vi "ShootAndTransfer5.vi"() -> ()   [LabVIEW 2010]
uses:
  EDSDK-Labview.llb/kEdsObjectEvents.ctl
  EDSDK-Labview.llb/LVuserEventForEDS.ctl
  EDSDK-Labview.llb/kEdsImageSrcs.ctl
  EDSDK-Labview.llb/EdsImageInfo.ctl
  EDSDK-Labview.llb/kEdsProperties.ctl
  EDSDK-Labview.llb/kEdsCameraStatusCommands.ctl
  EDSDK-Labview.llb/kEdsCameraCommands.ctl
  kernel32.dll
  EDSDK-Labview.llb/kEdsCameraCommand_ShutterButton.ctl
panel:
  out "images to download":i32
  out "images to decode":i32
  out "dt download":u32[](array[numeric])
  out "delay from shoot":u32[](array[numeric])
  out "dt decode":u32[](array[numeric])
  out "total decode cycle":u32
  out "body ids":u32[](array[numeric])
  out "ref":u32
  out "grab error out":errorcluster
  out "shoot error out":errorcluster
  in  "shoot cycle duration":u32=4000
  out "images":T1[](array[plugin-control])
  out "shoot #":i32
  out "event":T2 items=["All"=512, "VolumeInfoChanged"=513, "VolumeUpdateItems"=514, "FolderUpdateItems"=515, "DirItemCreated"=516, "DirItemRemoved"=517, "DirItemInfoChanged"=518, "DirItemContentChanged"=519, "DirItemRequestTransfer"=520, "DirItemRequestTransferDT"=521, "DirItemCancelTransferDT"=522, "VolumeAdded"=524, "VolumeRemoved"=525]
  in  "Image Type":T3=4 items=["Grayscale (U8)", "Grayscale (I16)", "Grayscale (SGL)", "Complex (CSG)", "RGB (U32)", "HSL (U32)", "RGB (U64)", "Grayscale (U16)"]
  in  "stop":bool
  out "cameras":u32
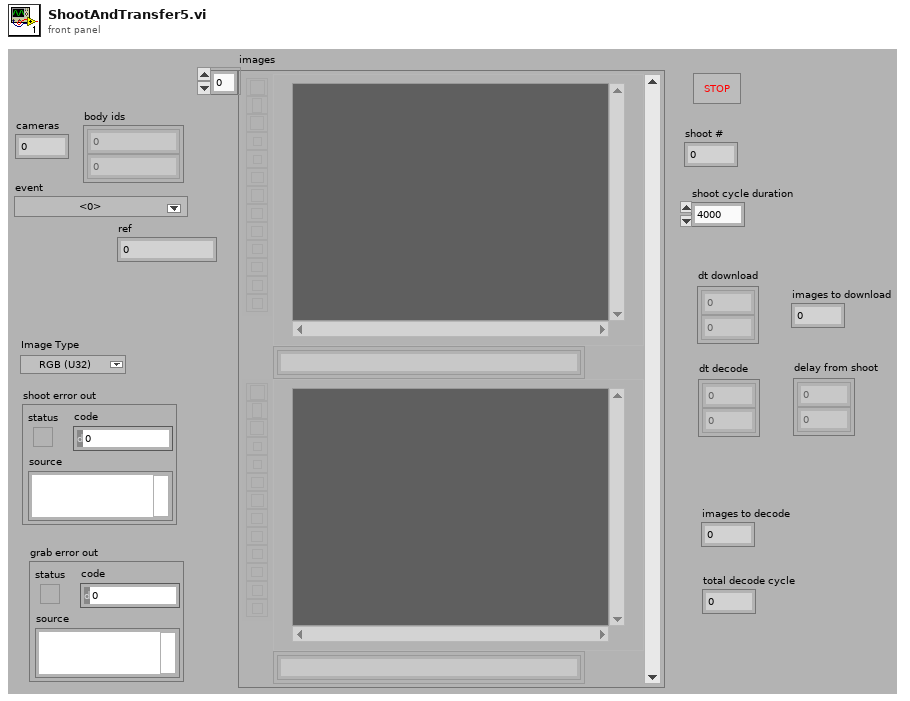
[diagram p1: front panel]
types:
  T1 = typedef "IMAQ Image.ctl" = refnum<image>
  T2 = typedef "kEdsObjectEvents.ctl" = u32
  T3 = typedef "Image Type" = u32
  T4 = typedef "LVuserEventForEDS.ctl" = cluster{"LVUserEventRef":u32, "event":u32, "ref":u32}
  T5 = typedef "kEdsImageSrcs.ctl" = u32
  T6 = typedef "EdsImageInfo.ctl" = cluster{"width":u32, "height":u32, "# components":u32, "bit depth":u32, "rect":u32[], "reserved 1":u32, "reserved 2":u32}
  T7 = cluster{"time Request":u32, "time downloaded":u32, "ImageRef":u32, "ImageSource":T5, "StreamRef":u32, "ImageInfo":T6}
  T8 = cluster{"numberOfFreeClusters":i32, "numberOfFreeSectors":i32, "reset":bool}
  T9 = typedef "kEdsProperties.ctl" = u32
  T10 = typedef "kEdsCameraCommands.ctl" = u32
  T11 = typedef "kEdsCameraCommand_ShutterButton.ctl" = u32
  T12 = cluster{"time":u32, "timer after download":u32, "ImageRef":u32, "ImageSource":T5, "outStreamRef":u32, "outImageInfo":T6}
  T13 = typedef "kEdsCameraStatusCommands.ctl" = u32
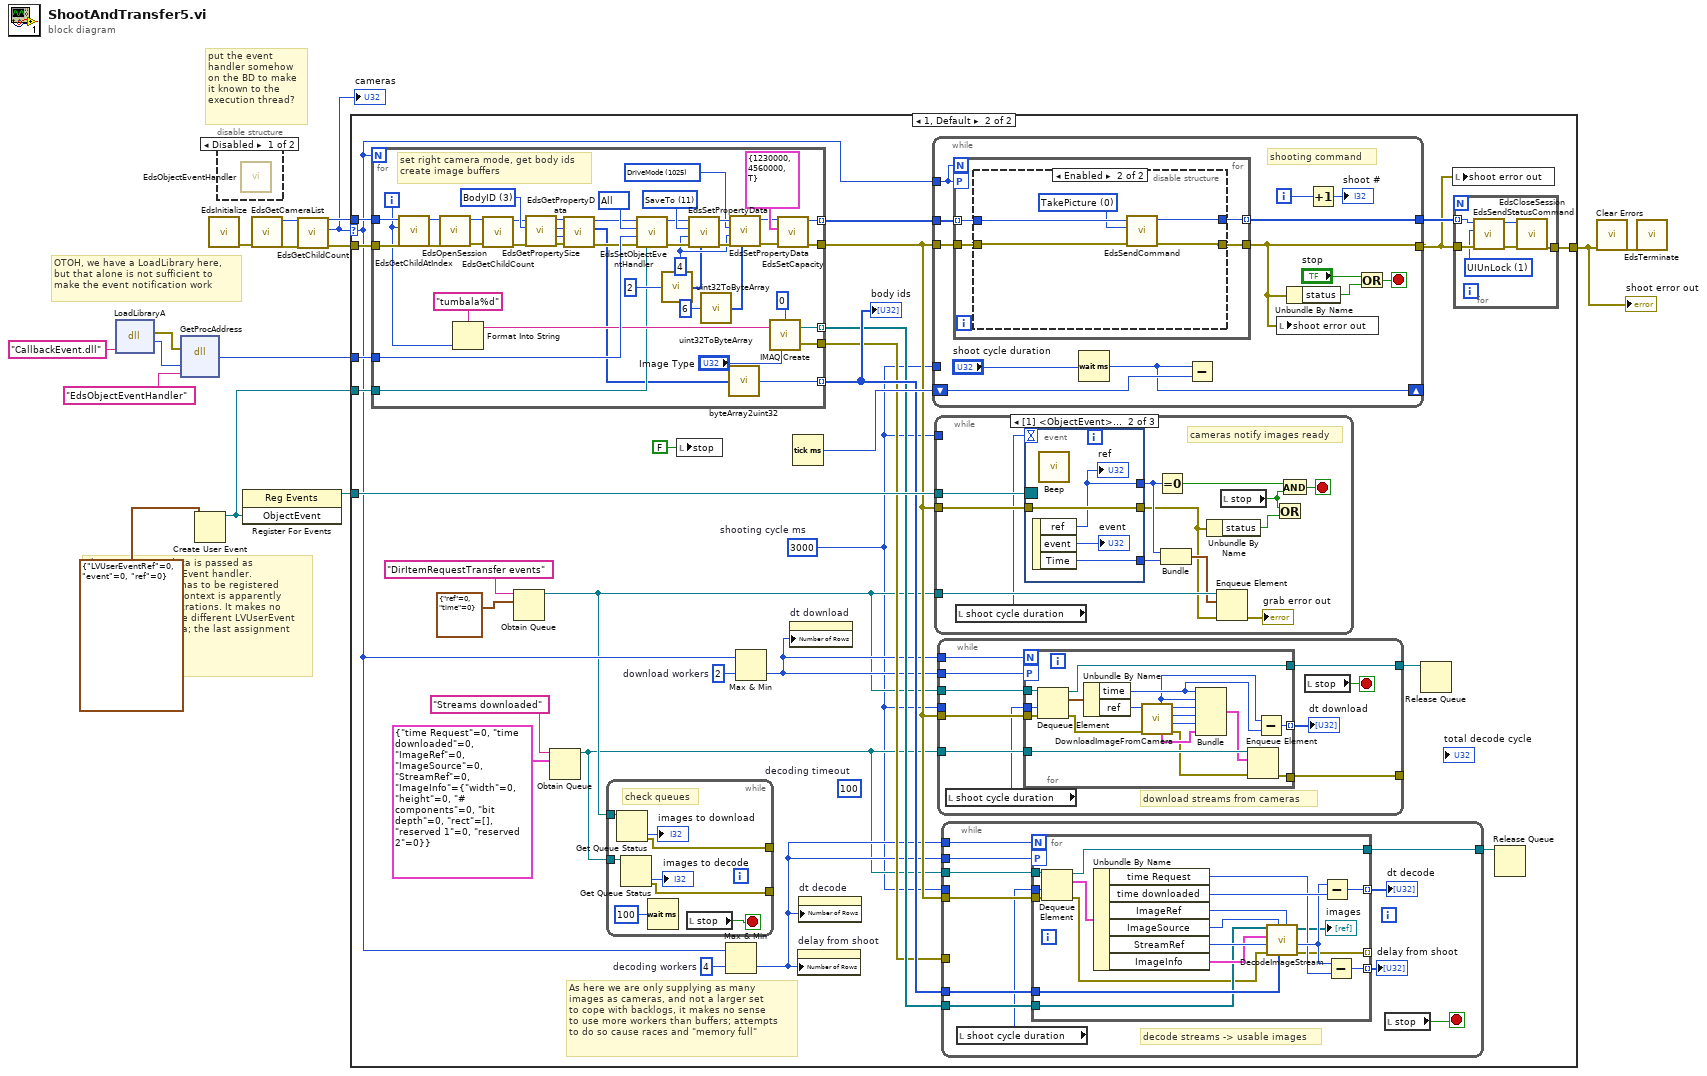
[diagram p0: block diagram]
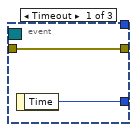
[diagram p4: hidden frame]
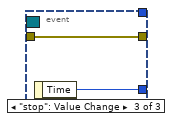
[diagram p5: hidden frame]
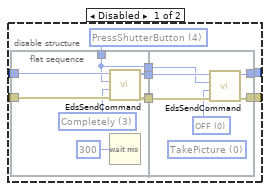
[diagram p6: hidden frame]
diagram:
  # "The LVUserEvent data is passed as \nInContext to EDSSetEvent handler.\nEven if the callback has to be registered\nfor each camera, InContext is apparently\ncommon to all registrations. It makes no\nsense to try to define different LVUserEvent\ndata for each camera; the last assignment\nrules."
  # "OTOH, we have a LoadLibrary here,\nbut that alone is not sufficient to\nmake the event notification work"
  # "put the event\nhandler somehow\non the BD to make\nit known to the\nexecution thread?"
  n1 = dll-call lib="kernel32.dll" fn="LoadLibraryA"("libraryName"="CallbackEvent.dll") -> (error out=w7:errorcluster, "return type"=w10:u32)  [unwired: 4 in, 1 out]
  n2 = dll-call lib="kernel32.dll" fn="GetProcAddress"(error in=w7, "address"=w10, "procName"="EdsObjectEventHandler") -> ("return type"=w8:u32)  [unwired: 4 in, 2 out]
  n3 = Create User Event(user event datatype=T4 {"LVUserEventRef"=0, "event"=0, "ref"=0} ("ObjectEvent")) -> (user event=w2:refnum<user-event>)  [unwired: 1 in, 1 out]
  n4 = call "EdsInitialize.vi"() -> ("error out"=w5:errorcluster)  [unwired: 11 in]
  n5 = disable-structure shown="Disabled" {
    frame Disabled {
      n6 = call "EdsObjectEventHandler.vi"() -> ()  [unwired: 7 in, 2 out]
    }
    frame Enabled {
    }
  }
  n7 = register-events(w2) -> (reference out=w3:refnum<event-registration>)  [unwired: 2 in, 1 out]
  n8 = call "EdsGetCameraList.vi"("error in"=w5) -> ("error out"=w14:errorcluster, "outCameraListRef"=w1:u32)  [unwired: 9 in]
  n9 = call "EdsGetChildCount.vi"("error in"=w14, "inRef"=w1) -> ("error out"=w6:errorcluster, "count"=w12:u32, "inRef dup"=w13:u32)  [unwired: 7 in]
  "cameras" <- w12
  n10 = case shown="1, Default" w12 {
    selector: w12 -> [_ w23]
    tunnel: w13 -> [_ w46]
    tunnel: w6 -> [w17 w45]
    tunnel: [w17 w44] -> w15
    tunnel: w8 -> [_ w43]
    tunnel: w3 -> [_ w37]
    tunnel: w2 -> [_ w36]
    frame 0 {
    }
    frame 1, Default {
      (unwired) u32 100  # decoding timeout
      w24 = u32 2  # download workers
      w22 = u32 4  # decoding workers
      w18 = u32 3000  # shooting cycle ms
      # "As here we are only supplying as many\nimages as cameras, and not a larger set\nto cope with backlogs, it makes no sense\nto use more workers than buffers; attempts\nto do so cause races and \"memory full\""
      n11 = for {
        N: w23 -> [_]
        tunnel: w46 -> [w180]
        tunnel: w45 -> [w179]
        tunnel: [w174] -> w27 mode=indexing
        tunnel: [w173] -> w26
        tunnel: w43 -> [w170]
        tunnel: [w152] -> w39 mode=indexing
        tunnel: [w151] -> w31
        tunnel: w36 -> [w153]
        tunnel: [w140] -> w28 mode=indexing
        i -> [w156]
        w147 = T9 3 items=["Unknown"=65535, "ProductName"=2, "BodyID"=3, "OwnerName"=4, "MakerName"=5, "DateTime"=6, "FirmwareVersion"=7, "BatteryLevel"=8, "CFn"=9, "SaveTo"=11, "CurrentStorage"=12, "CurrentFolder"=13, "MyMenu"=14, "BatteryQuality"=16, "HDDirectoryStructure"=32, "ImageQuality"=256, "JpegQuality"=257, "Orientation"=258, "ICCProfile"=259, "FocusInfo"=260, "DigitalExposure"=261, "WhiteBalance"=262, "ColorTemperature"=263, "WhiteBalanceShift"=264, "Contrast"=265, "ColorSaturation"=266, "ColorTone"=267, "Sharpness"=268, "ColorSpace"=269, "ToneCurve"=270, "PhotoEffect"=271, "FilterEffect"=272, "ToningEffect"=273, "ParameterSet"=274, "ColorMatrix"=275, "PictureStyle"=276, "PictureStyleDesc"=277, "ETTL2Mode"=279, "PictureStyleCaption"=512, "Linear"=768, "ClickWBPoint"=769, "WBCoeffs"=770, "GPSVersionID"=2048, "GPSLatitudeRef"=2049, "GPSLatitude"=2050, "GPSLongitudeRef"=2051, "GPSLongitude"=2052, "GPSAltitudeRef"=2053, "GPSAltitude"=2054, "GPSTimeStamp"=2055, "GPSSatellites"=2056, "GPSStatus"=2057, "GPSMapDatum"=2066, "GPSDateStamp"=2077, "AtCapture_Flag"=2147483648, "AEMode"=1024, "DriveMode"=1025, "ISOSpeed"=1026, "MeteringMode"=1027, "AFMode"=1028, "Av"=1029, "Tv"=1030, "ExposureCompensation"=1031, "FlashCompensation"=1032, "FocalLength"=1033, "AvailableShots"=1034, "Bracket"=1035, "WhiteBalanceBracket"=1036, "LensName"=1037, "AEBracket"=1038, "FEBracket"=1039, "ISOBracket"=1040, "NoiseReduction"=1041, "FlashOn"=1042, "RedEye"=1043, "FlashMode"=1044, "LensStatus"=1046, "Artist"=1048, "Copyright"=1049, "DepthOfField"=1051, "EFCompensation"=1054, "Evf_OutputDevice"=1280, "Evf_Mode"=1281, "Evf_WhiteBalance"=1282, "Evf_ColorTemperature"=1283, "Evf_DepthOfFieldPreview"=1284, "Evf_Zoom"=1287, "Evf_ZoomPosition"=1288, "Evf_FocusAid"=1289, "Evf_Histogram"=1290, "Evf_ImagePosition"=1291, "Evf_HistogramStatus"=1292, "Evf_AFMode"=1294, "Evf_CoordinateSystem"=1344, "Evf_ZoomRect"=1345] ("inPropertyID")
        w161 = T9 1025 items=["Unknown"=65535, "ProductName"=2, "BodyID"=3, "OwnerName"=4, "MakerName"=5, "DateTime"=6, "FirmwareVersion"=7, "BatteryLevel"=8, "CFn"=9, "SaveTo"=11, "CurrentStorage"=12, "CurrentFolder"=13, "MyMenu"=14, "BatteryQuality"=16, "HDDirectoryStructure"=32, "ImageQuality"=256, "JpegQuality"=257, "Orientation"=258, "ICCProfile"=259, "FocusInfo"=260, "DigitalExposure"=261, "WhiteBalance"=262, "ColorTemperature"=263, "WhiteBalanceShift"=264, "Contrast"=265, "ColorSaturation"=266, "ColorTone"=267, "Sharpness"=268, "ColorSpace"=269, "ToneCurve"=270, "PhotoEffect"=271, "FilterEffect"=272, "ToningEffect"=273, "ParameterSet"=274, "ColorMatrix"=275, "PictureStyle"=276, "PictureStyleDesc"=277, "ETTL2Mode"=279, "PictureStyleCaption"=512, "Linear"=768, "ClickWBPoint"=769, "WBCoeffs"=770, "GPSVersionID"=2048, "GPSLatitudeRef"=2049, "GPSLatitude"=2050, "GPSLongitudeRef"=2051, "GPSLongitude"=2052, "GPSAltitudeRef"=2053, "GPSAltitude"=2054, "GPSTimeStamp"=2055, "GPSSatellites"=2056, "GPSStatus"=2057, "GPSMapDatum"=2066, "GPSDateStamp"=2077, "AtCapture_Flag"=2147483648, "AEMode"=1024, "DriveMode"=1025, "ISOSpeed"=1026, "MeteringMode"=1027, "AFMode"=1028, "Av"=1029, "Tv"=1030, "ExposureCompensation"=1031, "FlashCompensation"=1032, "FocalLength"=1033, "AvailableShots"=1034, "Bracket"=1035, "WhiteBalanceBracket"=1036, "LensName"=1037, "AEBracket"=1038, "FEBracket"=1039, "ISOBracket"=1040, "NoiseReduction"=1041, "FlashOn"=1042, "RedEye"=1043, "FlashMode"=1044, "LensStatus"=1046, "Artist"=1048, "Copyright"=1049, "DepthOfField"=1051, "EFCompensation"=1054, "Evf_OutputDevice"=1280, "Evf_Mode"=1281, "Evf_WhiteBalance"=1282, "Evf_ColorTemperature"=1283, "Evf_DepthOfFieldPreview"=1284, "Evf_Zoom"=1287, "Evf_ZoomPosition"=1288, "Evf_FocusAid"=1289, "Evf_Histogram"=1290, "Evf_ImagePosition"=1291, "Evf_HistogramStatus"=1292, "Evf_AFMode"=1294, "Evf_CoordinateSystem"=1344, "Evf_ZoomRect"=1345] ("inPropertyID")
        w171 = T2 512 items=["All"=512, "VolumeInfoChanged"=513, "VolumeUpdateItems"=514, "FolderUpdateItems"=515, "DirItemCreated"=516, "DirItemRemoved"=517, "DirItemInfoChanged"=518, "DirItemContentChanged"=519, "DirItemRequestTransfer"=520, "DirItemRequestTransferDT"=521, "DirItemCancelTransferDT"=522, "VolumeAdded"=524, "VolumeRemoved"=525] ("inEvent")
        w162 = u32 4 ("inPropertySize")
        w172 = T9 11 items=["Unknown"=65535, "ProductName"=2, "BodyID"=3, "OwnerName"=4, "MakerName"=5, "DateTime"=6, "FirmwareVersion"=7, "BatteryLevel"=8, "CFn"=9, "SaveTo"=11, "CurrentStorage"=12, "CurrentFolder"=13, "MyMenu"=14, "BatteryQuality"=16, "HDDirectoryStructure"=32, "ImageQuality"=256, "JpegQuality"=257, "Orientation"=258, "ICCProfile"=259, "FocusInfo"=260, "DigitalExposure"=261, "WhiteBalance"=262, "ColorTemperature"=263, "WhiteBalanceShift"=264, "Contrast"=265, "ColorSaturation"=266, "ColorTone"=267, "Sharpness"=268, "ColorSpace"=269, "ToneCurve"=270, "PhotoEffect"=271, "FilterEffect"=272, "ToningEffect"=273, "ParameterSet"=274, "ColorMatrix"=275, "PictureStyle"=276, "PictureStyleDesc"=277, "ETTL2Mode"=279, "PictureStyleCaption"=512, "Linear"=768, "ClickWBPoint"=769, "WBCoeffs"=770, "GPSVersionID"=2048, "GPSLatitudeRef"=2049, "GPSLatitude"=2050, "GPSLongitudeRef"=2051, "GPSLongitude"=2052, "GPSAltitudeRef"=2053, "GPSAltitude"=2054, "GPSTimeStamp"=2055, "GPSSatellites"=2056, "GPSStatus"=2057, "GPSMapDatum"=2066, "GPSDateStamp"=2077, "AtCapture_Flag"=2147483648, "AEMode"=1024, "DriveMode"=1025, "ISOSpeed"=1026, "MeteringMode"=1027, "AFMode"=1028, "Av"=1029, "Tv"=1030, "ExposureCompensation"=1031, "FlashCompensation"=1032, "FocalLength"=1033, "AvailableShots"=1034, "Bracket"=1035, "WhiteBalanceBracket"=1036, "LensName"=1037, "AEBracket"=1038, "FEBracket"=1039, "ISOBracket"=1040, "NoiseReduction"=1041, "FlashOn"=1042, "RedEye"=1043, "FlashMode"=1044, "LensStatus"=1046, "Artist"=1048, "Copyright"=1049, "DepthOfField"=1051, "EFCompensation"=1054, "Evf_OutputDevice"=1280, "Evf_Mode"=1281, "Evf_WhiteBalance"=1282, "Evf_ColorTemperature"=1283, "Evf_DepthOfFieldPreview"=1284, "Evf_Zoom"=1287, "Evf_ZoomPosition"=1288, "Evf_FocusAid"=1289, "Evf_Histogram"=1290, "Evf_ImagePosition"=1291, "Evf_HistogramStatus"=1292, "Evf_AFMode"=1294, "Evf_CoordinateSystem"=1344, "Evf_ZoomRect"=1345] ("inPropertyID")
        # "set right camera mode, get body ids\ncreate image buffers"
        n12 = call "EdsGetChildAtIndex.vi"("error in"=w179, "index"=w156, "inRef"=w180) -> ("error out"=w181:errorcluster, "outRef"=w182:u32)  [unwired: 7 in]
        n13 = call "EdsOpenSession.vi"("error in"=w181, "inCameraRef"=w182) -> ("error out"=w177:errorcluster, "inCameraRef dup"=w178:u32)  [unwired: 8 in]
        n14 = Format Into String(format string="tumbala%d" ("Image Name"), w156) -> (resulting string=w154:string)  [unwired: 2 in, 1 out]
        n15 = call "EdsGetChildCount.vi"("error in"=w177, "inRef"=w178) -> ("error out"=w145:errorcluster, "inRef dup"=w144:u32)  [unwired: 7 in, 1 out]
        n16 = call "EdsGetPropertySize.vi"("error in"=w145, "inPropertyID"=w147, "inRef"=w144) -> ("error out"=w149:errorcluster, "outSize"=w148:u32, "inPropertyID dup"=w150:T9, "inRef dup"=w146:u32)  [unwired: 4 in, 1 out]
        n17 = call "EdsGetPropertyData.vi"("error in"=w149, "inPropertySize"=w148, "inPropertyID"=w150, "inRef"=w146) -> ("error out"=w143:errorcluster, "outPropertyData"=w141:u8[], "inRef dup"=w142:u32)  [unwired: 5 in]
        n18 = call "EdsSetObjectEventHandler.vi"("user event out"=w153, "error in"=w143, "inObjectEventHandler"=w170, "inEvent"=w171, "inCameraRef"=w142) -> ("error out"=w169:errorcluster, "inCameraRef dup"=w168:u32)  [unwired: 2 in]
        n19 = call "uint32ToByteArray.vi"("Numeric"=u32 2) -> ("inPropertyData"=w160:u8[])  [unwired: 4 in]
        n20 = call "EdsSetPropertyData.vi"("inPropertyData"=w160, "error in"=w169, "inPropertySize"=w162, "inPropertyID"=w172, "inRef"=w168) -> ("error out"=w166:errorcluster, "inRef dup"=w165:u32)  [unwired: 5 in]
        n21 = call "uint32ToByteArray.vi"("Numeric"=u32 6) -> ("inPropertyData"=w158:u8[])  [unwired: 4 in]
        n22 = call "byteArray2uint32.vi"("byteArray"=w141) -> ("uint32"=w140:u32)
        n23 = call "EdsSetPropertyData.vi"("inPropertyData"=w158, "error in"=w166, "inPropertySize"=w162, "inPropertyID"=w161, "inRef"=w165) -> ("error out"=w164:errorcluster, "inRef dup"=w163:u32)  [unwired: 5 in]
        n24 = call "IMAQ Create"("Border Size"=0, "Image Name"=w154, "Image Type"="Image Type") -> ("New Image"=w174:T1, "error out"=w173:errorcluster)  [unwired: 2 in]
        n25 = call "EdsSetCapacity.vi"("error in"=w164, "inCapacity"=T8 {"numberOfFreeClusters"=1230000, "numberOfFreeSectors"=4560000, "reset"=TRUE}, "inCameraRef"=w163) -> ("error out"=w151:errorcluster, "inCameraRef dup"=w152:u32)  [unwired: 7 in]
      }
      "body ids" <- w28
      n26 = Obtain Queue(name (unnamed)="DirItemRequestTransfer events", element data type=cluster{"ref":u32, "time":u32} {"ref"=0, "time"=0}) -> (queue out=w20:refnum<queue>)  [unwired: 3 in, 2 out]
      n27 = Obtain Queue(name (unnamed)="Streams downloaded", element data type=T7 {"time Request"=0, "time downloaded"=0, "ImageRef"=0, "ImageSource"=0, "StreamRef"=0, "ImageInfo"={"width"=0, "height"=0, "# components"=0, "bit depth"=0, "rect"=[], "reserved 1"=0, "reserved 2"=0}}) -> (queue out=w19:refnum<queue>)  [unwired: 3 in, 2 out]
      n28 = while {
        tunnel: w20 -> [w50]
        tunnel: w19 -> [w49]
        tunnel: [w48] -> _
        tunnel: [w47] -> _
        stop <- w53 stop-if-true
        # "check queues"
        n29 = Get Queue Status(queue=w50) -> (error out=w48:errorcluster, # elements in queue=→"images to download":i32)  [unwired: 2 in, 6 out]
        n30 = Get Queue Status(queue=w49) -> (error out=w47:errorcluster, # elements in queue=→"images to decode":i32)  [unwired: 2 in, 6 out]
        n31 = Wait (ms)(milliseconds to wait=u32 100) -> ()  [unwired: 1 out]
        n32 = local read "stop"() -> (w53:bool)
      }
      n33 = local write "stop"(FALSE ("stop")) -> ()
      n34 = Max & Min(x=w23, y=w22) -> (min(x,y)=w21:u32)  [unwired: 1 out]
      n35 = Max & Min(x=w23, y=w24) -> (min(x,y)=w25:u32)  [unwired: 1 out]
      n36 = property on="dt download" class="Arr (strict)"("Number of Rows"=w25) -> ()  [unwired: 2 in, 2 out]
      n37 = Tick Count (ms)() -> (millisecond timer value=w40:u32)
      n38 = property on="delay from shoot" class="Arr (strict)"("Number of Rows"=w21) -> ()  [unwired: 2 in, 2 out]
      n39 = property on="dt decode" class="Arr (strict)"("Number of Rows"=w21) -> ()  [unwired: 2 in, 2 out]
      n40 = while {
        tunnel: w31 -> [w195]
        tunnel: [w186] -> w38
        shift-right: [w184] -> _
        shift-left: w40 -> [w187]
        tunnel: w39 -> [w194]
        tunnel: [w190] -> w42
        tunnel: w23 -> [w185]
        tunnel: w18 -> [_]
        i -> [w188]
        stop <- w193 stop-if-true
        # "shooting command"
        n41 = for {
          N: w185 -> [_]
          tunnel: w195 -> [w199]
          tunnel: w194 -> [w198] mode=indexing
          tunnel: [w197] -> w190 mode=indexing
          tunnel: [w196] -> w186
          workers-P: w185 -> [_]
          n42 = disable-structure shown="Enabled" {
            disable-tunnel: w199 -> [w204 w225]
            disable-tunnel: w198 -> [w203 w224]
            disable-tunnel: [w201 w226] -> w196
            disable-tunnel: [w200 w227] -> w197
            frame Disabled {
              w202 = T10 4 items=["TakePicture"=0, "ExtendShutDownTimer"=1, "BulbStart"=2, "BulbEnd"=3, "DoEvfAf"=258, "DriveLensEvf"=259, "DoClickWBEvf"=260, "PressShutterButton"=4] ("inCommand")
              n43 = flat-sequence {
                tunnel: w204 -> [w216]
                tunnel: w203 -> [w215]
                tunnel: w202 -> [w211]
                tunnel: [w213] -> w209
                tunnel: [w212] -> w208
                tunnel: [w213] -> w207
                tunnel: [w212] -> w206
                tunnel: [w211] -> w205
                tunnel: [w220] -> w200
                tunnel: [w219] -> w201
                tunnel: w209 -> [_]
                tunnel: w208 -> [_]
                tunnel: w207 -> [w222]
                tunnel: w206 -> [w221]
                tunnel: w205 -> [w218]
                frame #0 {
                  w214 = T11 3 items=["OFF"=0, "Halfway"=1, "Completely"=3, "Halfway_NonAF"=65537, "Completely_NonAF"=65539] ("ShutterButton")
                  n44 = call "EdsSendCommand.vi"("error in"=w216, "inParam"=w214, "inCommand"=w211, "inRef"=w215) -> ("error out"=w213:errorcluster, "inRef dup"=w212:u32)  [unwired: 2 in]
                  n45 = Wait (ms)(milliseconds to wait=u32 300) -> ()  [unwired: 1 out]
                }
                frame #1 {
                  (unwired) T10 0 items=["TakePicture"=0, "ExtendShutDownTimer"=1, "BulbStart"=2, "BulbEnd"=3, "DoEvfAf"=258, "DriveLensEvf"=259, "DoClickWBEvf"=260, "PressShutterButton"=4] ("inCommand")
                  w217 = T11 0 items=["OFF"=0, "Halfway"=1, "Completely"=3, "Halfway_NonAF"=65537, "Completely_NonAF"=65539] ("ShutterButton")
                  n46 = call "EdsSendCommand.vi"("error in"=w222, "inParam"=w217, "inCommand"=w218, "inRef"=w221) -> ("error out"=w219:errorcluster, "inRef dup"=w220:u32)  [unwired: 2 in]
                }
              }
            }
            frame Enabled {
              w223 = T10 0 items=["TakePicture"=0, "ExtendShutDownTimer"=1, "BulbStart"=2, "BulbEnd"=3, "DoEvfAf"=258, "DriveLensEvf"=259, "DoClickWBEvf"=260, "PressShutterButton"=4] ("inCommand")
              n47 = call "EdsSendCommand.vi"("error in"=w225, "inCommand"=w223, "inRef"=w224) -> ("error out"=w226:errorcluster, "inRef dup"=w227:u32)  [unwired: 3 in]
            }
          }
        }
        n48 = Wait (ms)(milliseconds to wait="shoot cycle duration") -> (millisecond timer value=w184:u32)
        n49 = Subtract(x=w184, y=w187) -> ()  [unwired: 1 out]
        n50 = local write "shoot error out"(w186) -> ()
        n51 = Unbundle By Name(w186) -> ("status"=w192:bool)
        n52 = Increment(x=w188) -> (x+1=→"shoot #":i32)
        n53 = Or(x="stop", y=w192) -> (x .or. y?=w193:bool)
      }
      n54 = while {
        tunnel: w37 -> [w123]
        tunnel: w31 -> [w124]
        tunnel: w18 -> [_]
        tunnel: w20 -> [w119]
        stop <- w121 stop-if-true
        # "cameras notify images ready"
        n55 = local read "shoot cycle duration"() -> (w113:u32)
        n56 = event shown="[1] <ObjectEvent>: User Event" {
          selector: w123 -> [_ _ _]
          dyn-events: _ -> [_ _ _]
          timeout: w113 -> [_ _ _]
          tunnel: w124 -> [w126 w131 w133]
          tunnel: [_ w130 _] -> w117
          tunnel: [w126 w131 w133] -> w115
          tunnel: [w127 w129 w132] -> w118
          event Timeout {
            n57 = event-data() -> ("Time"=w127:u32)  [unwired: 1 in]
          }
          event User Event {
            n58 = event-data() -> ("ref"=w130:u32, "event"=→"event":u32, "Time"=w129:u32)  [unwired: 1 in]
            "ref" <- w130
            n59 = call <vilib>:"Beep.vi"() -> ()  [unwired: 12 in]
          }
          event "stop": Value Change {
            n60 = event-data() -> ("Time"=w132:u32)  [unwired: 1 in]
          }
        }
        n61 = Equal To 0?(x=w117) -> (x = 0?=w120:bool)
        n62 = Bundle("ref"=w117, "Time"=w118) -> (w116:cluster{"ref":u32, "Time":u32})  [unwired: 1 in]
        n63 = Unbundle By Name(w115) -> ("status"=w125:bool)
        n64 = Enqueue Element(queue=w119, element=w116, error in (no error)=w115) -> (error out=→"grab error out":errorcluster)  [unwired: 1 in, 2 out]
        n65 = local read "stop"() -> (w122:bool)
        n66 = Or(x=w122, y=w125) -> ()  [unwired: 1 out]
        n67 = And(x=w120, y=w122) -> (x .and. y?=w121:bool)
      }
      n68 = while {
        tunnel: w20 -> [w94]
        tunnel: w18 -> [_]
        tunnel: w31 -> [w91]
        tunnel: w19 -> [w92]
        tunnel: [w86] -> w30
        tunnel: [w90] -> _
        tunnel: w25 -> [w89]
        tunnel: w25 -> [w88]
        stop <- w93 stop-if-true
        # "download streams from cameras"
        n69 = local read "shoot cycle duration"() -> (w85:u32)
        n70 = for {
          N: w88 -> [_]
          tunnel: w94 -> [w112]
          tunnel: w85 -> [w111]
          tunnel: w92 -> [w104]
          tunnel: [w102] -> w86
          tunnel: w91 -> [w101]
          tunnel: [w98] -> w87 mode=indexing
          tunnel: [w95] -> w90
          workers-P: w89 -> [_]
          n71 = Dequeue Element(queue=w112, timeout in ms (-1)=w111, error in (no error)=w101) -> (queue out=w102:refnum<queue>, element=w110:cluster{"ref":u32, "time":u32}, error out=w100:errorcluster)  [unwired: 1 out]
          n72 = Unbundle By Name(w110) -> ("time"=w97:u32, "ref"=w109:u32)
          n73 = call "DownloadImageFromCamera.vi"("error in"=w100, "dirItemRef in"=w109) -> ("outImageInfo"=w105:T6, "timer after download"=w96:u32, "error out"=w99:errorcluster, "outStreamRef"=w106:u32, "ImageSource"=w107:T5, "ImageRef"=w108:u32)  [unwired: 2 in]
          n74 = Bundle("time"=w97, "timer after download"=w96, "ImageRef"=w108, "ImageSource"=w107, "outStreamRef"=w106, "outImageInfo"=w105) -> (w103:T12)  [unwired: 1 in]
          n75 = Enqueue Element(queue=w104, element=w103, error in (no error)=w99) -> (error out=w95:errorcluster)  [unwired: 1 in, 2 out]
          n76 = Subtract(x=w96, y=w97) -> (x-y=w98:u32)
        }
        "dt download" <- w87
        n77 = local read "stop"() -> (w93:bool)
      }
      n78 = while {
        tunnel: w19 -> [w57]
        tunnel: w18 -> [_]
        tunnel: w31 -> [w62]
        tunnel: [w56] -> w29
        tunnel: w28 -> [w64]
        tunnel: w27 -> [w63]
        tunnel: w26 -> [_]
        tunnel: w21 -> [w61]
        tunnel: w21 -> [w58]
        stop <- w65 stop-if-true
        # "decode streams -> usable images"
        n79 = local read "shoot cycle duration"() -> (w55:u32)
        n80 = for {
          N: w61 -> [_]
          tunnel: w57 -> [w84]
          tunnel: w55 -> [w83]
          tunnel: [w81] -> w56
          tunnel: w64 -> [w78]
          tunnel: w63 -> [w77]
          tunnel: w62 -> [w75]
          tunnel: [w72] -> w60 mode=indexing
          tunnel: [w70] -> w59 mode=indexing
          workers-P: w58 -> [_]
          tunnel: [w67] -> _ mode=indexing
          n81 = Dequeue Element(queue=w84, timeout in ms (-1)=w83, error in (no error)=w75) -> (queue out=w81:refnum<queue>, element=w82:T7, error out=w74:errorcluster)  [unwired: 1 out]
          n82 = Unbundle By Name(w82) -> ("time Request"=w68:u32, "time downloaded"=w71:u32, "ImageRef"=w76:u32, "ImageSource"=w73:T5, "StreamRef"=w80:u32, "ImageInfo"=w79:T6)
          n83 = call "DecodeImageStream.vi"("ImageRef"=w76, "Camera body ids"=w78, "ImageSource"=w73, "error in"=w74, "StreamRef"=w80, "ImageInfo"=w79, "Images array"=w77) -> ("error out"=w67:errorcluster, "timer after decoding"=w69:u32, "Image Array out"=→"images":T1[])  [unwired: 2 in]
          n84 = Subtract(x=w69, y=w71) -> (x-y=w72:u32)
          n85 = Subtract(x=w69, y=w68) -> (x-y=w70:u32)
        }
        "dt decode" <- w60
        "delay from shoot" <- w59
        n86 = local read "stop"() -> (w65:bool)
      }
      n87 = Release Queue(queue=w30) -> ()  [unwired: 2 in, 3 out]
      n88 = local write "shoot error out"(w38) -> ()
      n89 = for {
        tunnel: [w139] -> w44
        tunnel: w42 -> [w138] mode=indexing
        tunnel: w38 -> [w136]
        w134 = T13 1 items=["UILock", "UIUnLock", "EnterDirectTransfer", "ExitDirectTransfer"] ("inCommand")
        n90 = call "EdsSendStatusCommand.vi"("error in"=w136, "inCommand"=w134, "inCameraRef"=w138) -> ("error out"=w135:errorcluster, "inCameraRef dup"=w137:u32)  [unwired: 3 in]
        n91 = call "EdsCloseSession.vi"("error in"=w135, "inCameraRef"=w137) -> ("error out"=w139:errorcluster)  [unwired: 8 in, 1 out]
      }
      n92 = Release Queue(queue=w29) -> ()  [unwired: 2 in, 3 out]
    }
  }
  "shoot error out" <- w15
  n93 = call <vilib>:"Clear Errors.vi"("error in (no error)"=w15) -> ("error out"=w16:errorcluster)  [unwired: 6 in]
  n94 = call "EdsTerminate.vi"("error in"=w16) -> ()  [unwired: 10 in, 1 out]
